vi "Main.vi"() -> ()   [LabVIEW 2020]
doc: "This template is for the Queued Message Handler design pattern.\n\nThe Event Handling Loop generates messages based on user interface actions.\n\nThe Message Handling Loop processes messages generated by the Event Handling Loop, or by other messages. The messages are string values, so new messages can be added easily to the Message Cases case structure in the Message Handling Loop. Each message cluster can also provide an optional value for Message Data, which is a variant that can be converted to whatever message-specific data is required."
uses:
  Newport_FCR100/Libraries/FCR100/Support/Device state -- enum.ctl
  controls/Analysis results -- cluster.ctl
  controls/Abeles-Brewster - Newport UI Data.ctl
  controls/DAQ config parameters -- cluster.ctl
  controls/FCR config parameters -- cluster.ctl
  support/Message Queue/Enqueue Message (Single).vi
  <vilib>/Utility/error.llb/Error Cluster From Error Code.vi
  <vilib>/ErrorRing/Error Ring.xnode
  support/Message Queue/Abeles-Brewster - Newport Message Queue.lvlib
  support/User Event - Stop/Abeles-Brewster - Newport User Event - Stop.lvlib
  Newport_FCR100/Libraries/FCR100/FCR100.lvlib
  NI_DAQ/Libraries/NI DAQ/NI DAQ.lvlib
panel:
  out "Auto?":bool
  out "State 2":T1=enum."Configuration" caption="FCR 2 state"
  out "State 1":T1=enum."Configuration" caption="FCR 1 State"
  out "FCR Connected":bool
  out "DAQ Connected":bool
  in  "Settings":bool
  out "Elapsed time":dbl
  in  "Velocity":dbl=6.0 min=0.001 max=15.0 step=0.001
  in  "Refresh":bool
  in  "Tab Control":T2(tab)
  out "Sensor Value":dbl(slide) caption="Sensor\nValue" scale=0.0..12.0
  out "Angle chart":cluster{"Angle":dbl, "Data":dbl}[](graph)
  in  "Save Data":bool
  in  "File name":string="dato"
  out "Time chart":cluster{"Angle":dbl, "Data":dbl}[](graph)
  in  "Start":bool
  in  "Test time":dbl=6.0
  out "SPR Curve":cluster{"Angle":dbl, "Data":dbl}[](graph)
  in  "q Starting":dbl=40.0 format="%#_g°"
  in  "q Final":dbl=70.0 format="%#_g°"
  in  "Open File":path
  in  "Realizar Análisis":bool
  out "No. de datos":i32
  out "Analysis results":T3 {"Curve width" format="%#.3g°"; "Maximum Intensity" format="%#_gV"; "q Middle" format="%#_g°"; "Minimum Intensity" format="%#_gV"; "qR" format="%#_g°"}
  out "Max":dbl format="%#_g°"
  out "Min":dbl format="%#_g°"
  out "elapsed time 2":dbl
  out "Curr angle":dbl caption="Current Angle P1" format="%#_g°"
  in  "Controls":T4={"AutoMove"={"Move"=FALSE, "Cancel"=FALSE, "Home"=FALSE, "Final Angle P1"=90.0, "Ángulo Final M2"=180.0}, "ManMove"={"Inc platina 1"=FALSE, "Dec platina 1"=FALSE, "Inc platina 2"=FALSE, "Dec platina 2"=FALSE, "Resolution"=1.0}} {"ManMove"."Resolution" min=0.0 max=60.0 step=0.001 format="%#_g°/mov"; "AutoMove"."Ángulo Final M2" min=0.0 max=200.0 step=0.001; "AutoMove"."Final Angle P1" min=0.0 max=250.0 step=0.001 format="%#_g°"}
  in  "Initial Angle P2":dbl=12.0 min=0.0 max=90.0 step=0.001 format="%#_g°"
  in  "Initial Angle P1":dbl=30.0 min=0.0 max=90.0 step=0.001 format="%#_g°"
  in  "Aceleration":dbl=100.0 min=0.001 max=200.0 step=0.001
  in  "Exit":bool
  out "Status":string
  # "CENTRO DE INVESTIGACIONES EN ÓPTICA\nPROGRAM: \nDUAL  STEPPER MOTOR STAGE CONTROL  \n\nDEVELOPMENT BY: M.O. DIEGO TORRES ARMENTA"
  # "q Range"
  # "Conexión platinas\nPlatina 1 -> inf (Dirección 1); Platina 2-> superior (Dirección 2)\nInterfaz USB - RS422-1.8  se cablea entre la computadora y el conector superior correspondiente de platina 1\nCable (azul) FC-CB1 se cablea del conector inferior de platina 1 al conector superior de platina 2.\nSe conectan los eliminadores o fuentes de voltaje a las platinas.\npor último debe de energizar las fuentes de voltaje.\n\n\nConexión tarjeta de adquisición y sensor\n\nConector de sensor-> Amarillo -12V, Rojo +12V, Negro referencia a tierra, Blanco señal.\n\nEl cable blanco del sensor debe ser cableado a la entrada A0 de la tarjeta de adquisición de datos DAQ\nLa DAQ debe ser conectada a la computadora por medio del cable USB correspondiente."
  # "CENTRO DE INVESTIGACIONES EN ÓPTICA\n\nInstrucciones de funcionamiento.\n\n1.- Primero debe asegurar que las conexiones están hechas de manera correcta. (ver apartado conexiones)\n     Platina inferior tiene dirección 1, platina superior tiene dirección 2.\n2.- Se selecciona la velocidad, aceleración, ángulo inicial platina 1 y ángulo inicial platina 2.\n3.- Se ejecuta el programa dando click en el ícono Run, en la parte superior izquierda.\n4.- Aparece una ventana para configurar la dirección de platina a la cual queremos conectarnos, en éste caso seleccionamos 1, además de que en dicha ventana debemos seleccionar la opción (), presionamos aceptar y se da inicio con la ejecución del programa.\n5.- Al ejecutar por primera ocación, plas platinas se moveran de manera automática a posición Home (0 grados), en ejecuciones posteriores se moverán al ángulo inicial predefinido de cada una de las platinas.\n6.- Para ajuste manual debe dar click en los botones Inc++ o Dec -- de cada una de las platinas, el movimiento se realizará la cantidad de grados configurados en el control Resolución, la resolución mínima es de 0.001 y la máxima es de 60, en caso de que las platinas estén en movimiento puede cancelarlo dando click en el botón Cancelar mov.\n7.- Puede mover en cualquier momento las platinas a posición Home (0 grados), presionando el botón Mover a Home.\n8.- Cuando realizó los ajustes necearios en cada platina, se procede a seleccionar el ángulo final de la platina 1,  aquí debe de verificar el ángulo actual de la platina 1  en el indicador correspondiente y debe sumar los grados que desea mover al ángulo actual.\n9.- Una vez configurado se procede a presionar el botón Mover y guardar, entonces las platinas comenzarán su movimiento, guardarán la información en un archivo el cual tiene como nombre la fecha y hora de ejecución del movimiento, adicionalmente se grafica la señal obtenida."
  # "P1"
  # "P2"
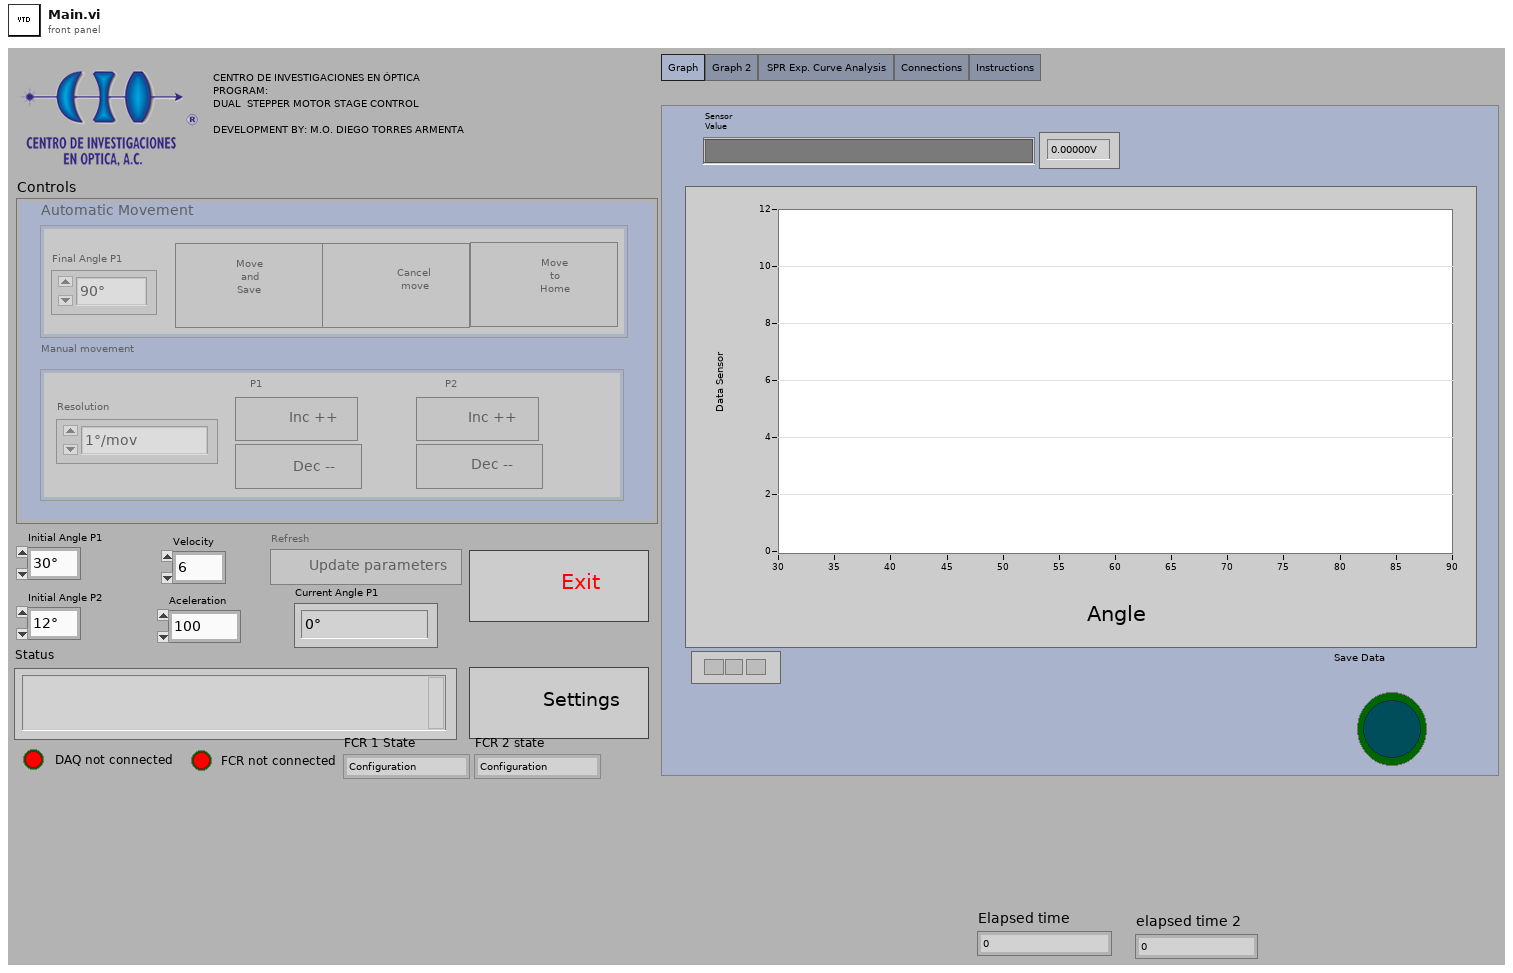
[diagram p1: front panel]
types:
  T1 = typedef "FCR100.lvlib/Device state -- enum.ctl" = enum16{"Not referenced", "Configuration", "Disable", "Ready", "Homing", "Motion"}
  T2 = enum32{"Graph", "Graph 2", "SPR Exp. Curve Analysis ", "Connections", "Instructions"}
  T3 = typedef "Analysis results -- cluster.ctl" = cluster{"q Middle":dbl, "Curve width":dbl, "Maximum Intensity":dbl, "Minimum Intensity":dbl, "qR ":dbl}
  T4 = cluster{"AutoMove":cluster{"Move":bool, "Cancel":bool, "Home":bool, "Final Angle P1":dbl, "Ángulo Final M2":dbl}, "ManMove":cluster{"Inc platina 1":bool, "Dec platina 1":bool, "Inc platina 2":bool, "Dec platina 2":bool, "Resolution":dbl}}
  T5 = typedef "Abeles-Brewster - Newport UI Data.ctl" = cluster{"FCR Mod ID":i32, "DAQ Mod ID":i32, "Status":string, "DAQ config params":T6, "FCR config params":T7, "Connected?":bool, "Home?":bool, "Device state 1":T1, "Device state 2":T1, "Time chart":cluster{"Angle":dbl, "Data":dbl}[], "Angle chart":cluster{"Angle":dbl, "Data":dbl}[], "Initial time":u32}
  T6 = typedef "DAQ config parameters -- cluster.ctl" = cluster{"DAQ Device Name":tag, "Physical channel":tag}
  T7 = typedef "FCR config parameters -- cluster.ctl" = cluster{"VISA resource":refnum<visa-resource-name>, "baud rate":u32, "Acceleration":dbl, "Velocity":dbl, "Initial P1":dbl, "Initial P2":dbl}
  T8 = typedef "FCR100.lvlib/Broadcast Events--cluster.ctl" = cluster{"Module Did Init":refnum<user-event>, "Status Updated":refnum<user-event>, "Error Reported":refnum<user-event>, "Module Did Stop":refnum<user-event>, "Update Module Execution Status":refnum<user-event>, "Device connected":refnum<user-event>, "Connection failed":refnum<user-event>, "Device disconnected":refnum<user-event>, "State reached":refnum<user-event>, "Home reached":refnum<user-event>}
  T9 = typedef "NI DAQ.lvlib/Broadcast Events--cluster.ctl" = cluster{"Module Did Init":refnum<user-event>, "Status Updated":refnum<user-event>, "Error Reported":refnum<user-event>, "Module Did Stop":refnum<user-event>, "Update Module Execution Status":refnum<user-event>, "Digital data acquired":refnum<user-event>, "Device connected":refnum<user-event>, "Connection failed":refnum<user-event>, "Analog data acquired":refnum<user-event>}
  T10 = typedef "Abeles-Brewster - Newport Message Queue.lvlib/All Message Queues.ctl" = cluster{"UI":refnum<queue>}
  T11 = enum8{"Enabled", "Disabled", "Disabled and Grayed Out"}
  T12 = enum16{"All", "DO task", "DI task", "AO task", "AI task"}
  T13 = cluster{"input terminal configuration":i32, "minimum value":dbl, "maximum value":dbl}
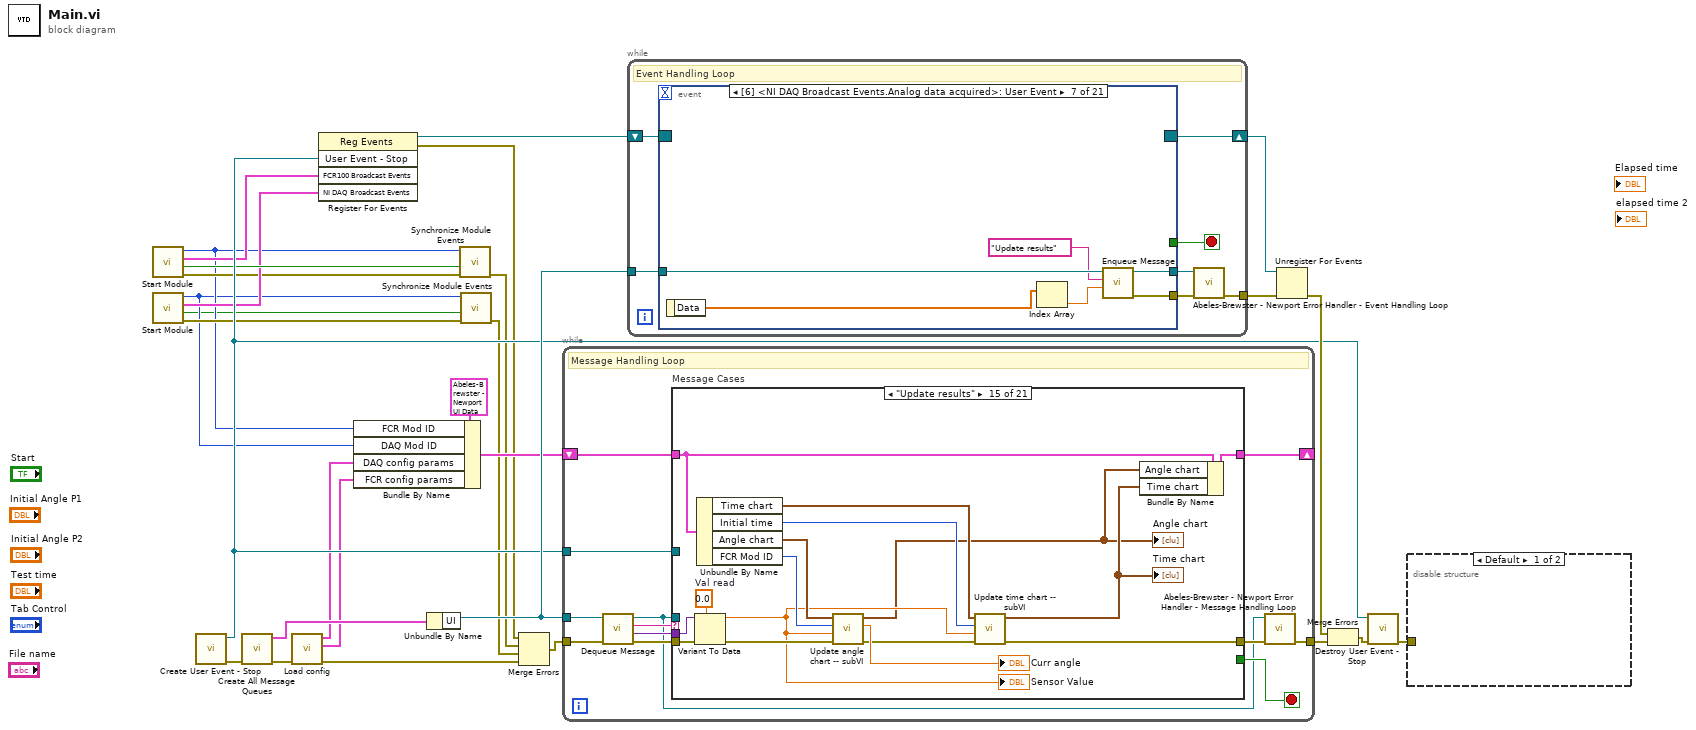
[diagram p0: block diagram]
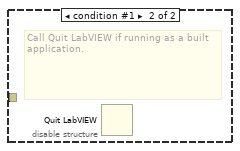
[diagram p2: hidden frame]
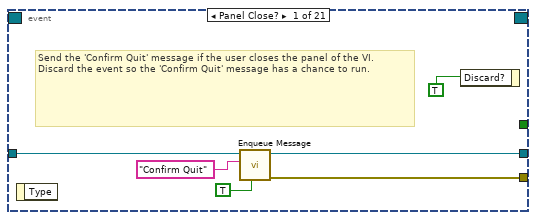
[diagram p3: hidden frame]
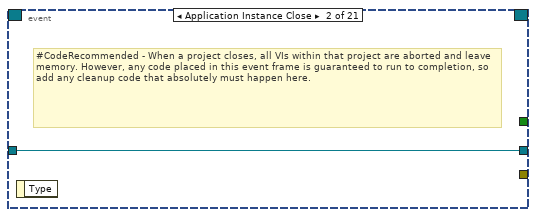
[diagram p4: hidden frame]
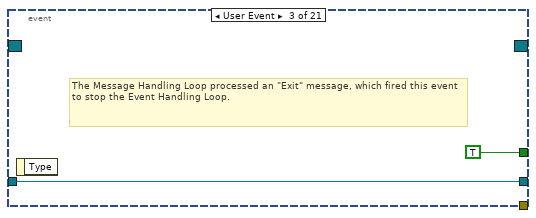
[diagram p5: hidden frame]
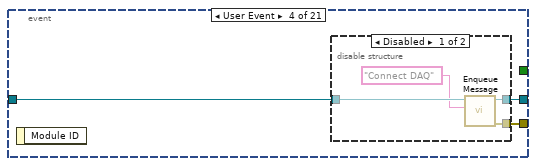
[diagram p6: hidden frame]
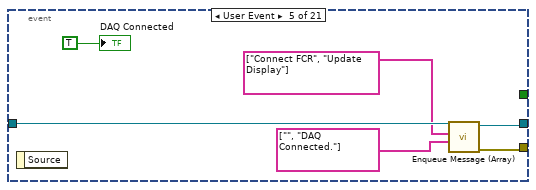
[diagram p8: hidden frame]
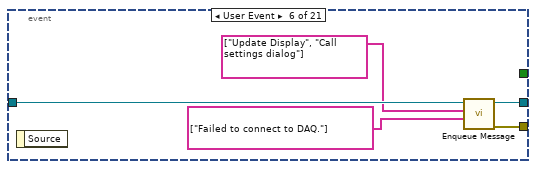
[diagram p9: hidden frame]
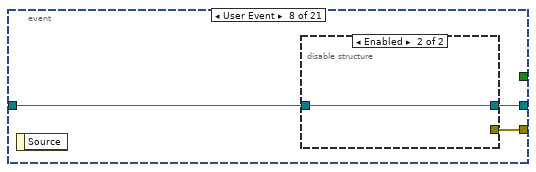
[diagram p10: hidden frame]
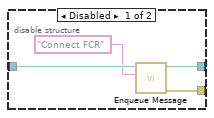
[diagram p11: hidden frame]
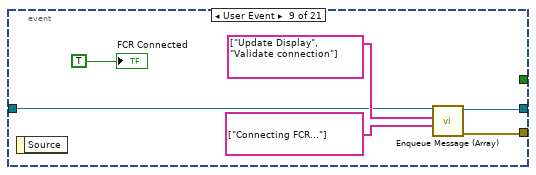
[diagram p12: hidden frame]
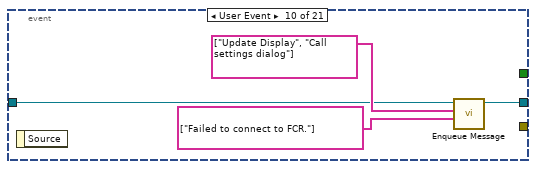
[diagram p13: hidden frame]
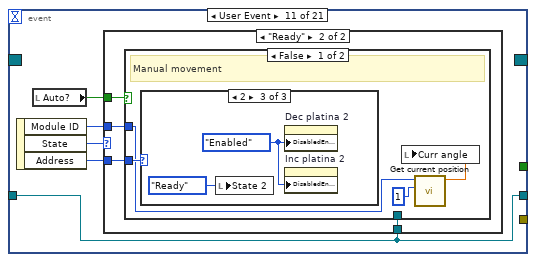
[diagram p14: hidden frame]
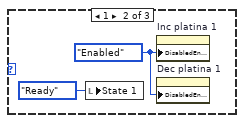
[diagram p17: hidden frame]
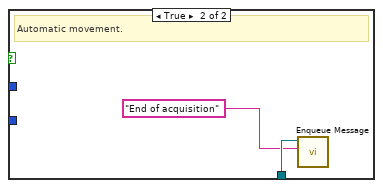
[diagram p18: hidden frame]
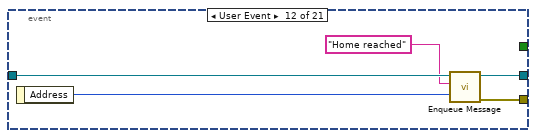
[diagram p19: hidden frame]
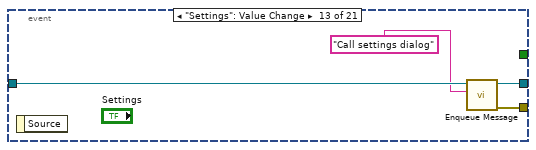
[diagram p20: hidden frame]
diagram:
  n1 = call "Start Module.vi"() -> ("error out"=w13:errorcluster, "Wait for Event Sync?"=w16:bool, "FCR100 Broadcast Events"=w17:T8, "Module ID"=w7:i32)  [unwired: 8 in]
  n2 = call "Start Module.vi"() -> ("error out"=w15:errorcluster, "Wait for Event Sync?"=w5:bool, "NI DAQ Broadcast Events"=w14:T9, "Module ID"=w6:i32)  [unwired: 8 in]
  n3 = call "Create User Event - Stop.vi"() -> ("error out"=w26:errorcluster, "User Event - Stop"=w19:refnum<user-event>)  [unwired: 10 in]
  n4 = call "Create All Message Queues.vi"("error in (no error)"=w26) -> ("error out"=w4:errorcluster, "Message Queues out"=w29:T10)  [unwired: 9 in]
  n5 = call "Load config.vi"("error in (no error)"=w4) -> ("DAQ config params"=w2:T6, "FCR config params"=w1:T7, "error out"=w3:errorcluster)  [unwired: 7 in]
  n6 = register-events(w19, w17, w14) -> (reference out=w20:refnum<event-registration>, error out=w8:errorcluster)  [unwired: 2 in]
  n7 = Bundle By Name(cluster=T5 {"FCR Mod ID"=0, "DAQ Mod ID"=0, "Status"="", "DAQ config params"={"DAQ Device Name"="Dev2", "Physical channel"=""}, "FCR config params"={"VISA resource"="", "baud rate"=9600, "Acceleration"=0.0, "Velocity"=0.0, "Initial P1"=0.0, "Initial P2"=0.0}, "Connected?"=FALSE, "Home?"=FALSE, "Device state 1"=enum."Configuration", "Device state 2"=enum."Configuration", "Time chart"=[], "Angle chart"=[], "Initial time"=0} ("Data Cluster"), "FCR Mod ID"=w7, "DAQ Mod ID"=w6, "DAQ config params"=w2, "FCR config params"=w1) -> (w11:T5)
  n8 = Unbundle By Name(w29) -> ("UI"=w27:refnum<queue>)
  n9 = call "Synchronize Module Events.vi"("error in"=w13, "Wait for Event Sync?"=w16, "Module ID in"=w7) -> ("error out"=w9:errorcluster)  [unwired: 7 in, 1 out]
  n10 = call "Synchronize Module Events.vi"("error in"=w15, "Wait for Event Sync?"=w5, "Module ID in"=w6) -> ("error out"=w10:errorcluster)  [unwired: 7 in, 1 out]
  n11 = Merge Errors(w8, w9, w10, w3) -> (w18:errorcluster)
  n12 = while {
    tunnel: w27 -> [w33]
    shift-right: [w40] -> _
    shift-left: w11 -> [w41]
    tunnel: w19 -> [w38]
    tunnel: w18 -> [w37]
    tunnel: [w32] -> w28
    stop <- w39 stop-if-true
    # "Message Handling Loop"
    n13 = call "Dequeue Message.vi"("error in (no error)"=w37, "Message Queue"=w33) -> ("error out"=w36:errorcluster, "Message Data"=w34:variant, "Message"=w35:string, "dup Message Queue"=w30:refnum<queue>)  [unwired: 6 in]
    n14 = case "Message Cases" shown="\"Update results\"" w35 {
      selector: w35 -> [_ _ _ _ _ _ _ _ _ _ _ _ _ _ _ _ _ _ _ _ w392]
      tunnel: w30 -> [w58 _ w84 w102 _ _ w125 _ w175 _ _ _ w270 w279 _ _ _ _ w363 w391 _]
      tunnel: w36 -> [w47 w76 w81 w105 w117 w123 w134 w160 w168 w180 w203 w258 w273 w285 w308 w323 w328 w360 w367 w386 _]
      tunnel: [w60 w77 w85 w104 w111 w122 w133 w158 w176 w185 w196 w256 w271 w282 w295 w311 w326 w354 w365 w389 w393] -> w31
      tunnel: w41 -> [w51 w63 w87 w106 w116 w121 w127 w153 w167 w184 w193 w249 w261 w284 w302 w324 w331 w359 w366 w382 w394]
      tunnel: [w50 w61 w89 w106 w116 w121 w126 w152 w174 w183 w192 w248 w259 w284 w301 w324 w331 w359 w366 w382 w394] -> w40
      tunnel: [_ _ _ _ _ _ _ _ _ _ _ _ _ _ _ _ _ _ _ TRUE _] -> w39
      tunnel: w34 -> [_ w75 _ _ _ _ _ _ _ _ w202 _ _ _ w306 w322 _ w358 _ w383 _]
      tunnel: w38 -> [_ _ _ _ _ _ _ _ _ _ _ _ _ _ _ _ _ _ _ w388 _]
      frame "Initialize" {
        w49 = FALSE ("Connected?")
        w56 = T11."Disabled and Grayed Out" ("Disabled")
        # "Initialize - All initialization work should take place in this message, since other loops can potentially enqueue messages that execute immediately after this one."
        n15 = control-ref of="This VI"() -> (w48:refnum<vi>)
        n16 = Unbundle By Name(w51) -> ("FCR config params.Acceleration"=w55:dbl, "FCR config params.Velocity"=w54:dbl, "FCR config params.Initial P1"=w53:dbl, "FCR config params.Initial P2"=w52:dbl)
        n17 = invoke on="Invoke Node" class="VI" method="Default Vals.Reinit All"(reference=w48, error in=w47) -> (reference out=w43:refnum<vi>, error out=w44:errorcluster)  [unwired: 1 in, 1 out]
        n18 = property on="Aceleration" class="DigNum (strict)"("Value"=w55) -> ()  [unwired: 2 in, 2 out]
        n19 = property on="Velocity" class="DigNum (strict)"("Value"=w54) -> ()  [unwired: 2 in, 2 out]
        n20 = property on="Initial P1" class="DigNum (strict)"("Value"=w53) -> ()  [unwired: 2 in, 2 out]
        n21 = property on="Initial P2" class="DigNum (strict)"("Value"=w52) -> ()  [unwired: 2 in, 2 out]
        n22 = invoke on="Invoke Node" class="VI" method="FP.Center"(reference=w43, error in=w44) -> (error out=w42:errorcluster)  [unwired: 1 in, 2 out]
        n23 = Bundle By Name(cluster=w51, "Connected?"=w49, "Home?"=w49, "Angle chart"=cluster{"Angle":dbl, "Data":dbl}[] [], "Time chart"=cluster{"Angle":dbl, "Data":dbl}[] []) -> (w50:T5)
        n24 = property on="AutoMove" class="Clust"("DisabledEnum"=w56) -> ()  [unwired: 2 in, 2 out]
        n25 = property on="ManMove" class="Clust"("DisabledEnum"=w56) -> ()  [unwired: 2 in, 2 out]
        n26 = property on="Refresh" class="Bool"("DisabledEnum"=w56) -> ()  [unwired: 2 in, 2 out]
        n27 = call-poly "Enqueue Message.vi"("error in (no error)"=w42, "Message Data Array"=string[] ["Initializing..."] ("Message"), "Message Array"=string[] ["Update Display", "Connect DAQ"] ("Message"), "Message Queue"=w58) -> ("error out"=w60:errorcluster)  [unwired: 6 in, 1 out]
      }
      frame "Update Display" {
        # "Update Display - Convert the message data to a string to display in the Data Display indicator."
        n28 = Variant To Data(error in=w76, type="", Variant=w75) -> (data=w68:string, error out=w66:errorcluster)
        n29 = Unbundle By Name(w63) -> ("Status"=w69:string)
        n30 = Get Date/Time In Seconds() -> (seconds since 1Jan1904=w72:timestamp)
        n31 = Format Date/Time String(time format string (%c)="%d/%m/%y %H:%M:%S%3u", seconds (now)=w72) -> (date/time string=w70:string)  [unwired: 1 in]
        n32 = Format Into String(format string="%s: %s\\n", initial string=w69, error in=w66, w70, w68) -> (resulting string=w62:string, error out=w67:errorcluster)
        "Status" <- w62
        n33 = property on="Status" class="Str"(error in=w67, "Text.Scroll Position"=u32 2000) -> (error out=w65:errorcluster)  [unwired: 1 in, 1 out]
        n34 = Bundle By Name(cluster=w63, "Status"=w62) -> (w61:T5)
        n35 = Merge Errors(w65) -> (w77:errorcluster)
      }
      frame "Call settings dialog" {
        n36 = Unbundle By Name(w87) -> ("DAQ config params"=w88:T6, "FCR config params"=w78:T7, "FCR Mod ID"=w80:i32)
        n37 = call "Disconnect.vi"("error in"=w81, "Module ID"=w80) -> ("error out"=w79:errorcluster)  [unwired: 9 in]
        n38 = call "Config dialog.vi"("error in (no error)"=w79, "FCR config params in"=w78, "DAQ config params in"=w88) -> ("error out"=w90:errorcluster, "Cancelled?"=w83:bool, "FCR config params out"=w82:T7, "DAQ config params out"=w86:T6)  [unwired: 5 in]
        n39 = case shown="False" w83 {
          tunnel: w90 -> [w94 w100]
          tunnel: w87 -> [w99 w101]
          tunnel: [w98 w101] -> w89
          tunnel: w86 -> [w92 _]
          tunnel: [w97 w100] -> w85
          tunnel: w84 -> [w96 _]
          tunnel: w82 -> [w91 _]
          frame False {
            # "Dialog not cancelled. Save and apply config."
            n40 = Bundle By Name(cluster=w99, "DAQ config params"=w92, "FCR config params"=w91) -> (w98:T5)
            n41 = call "Write config.vi"("error in (no error)"=w94, "FCR config params"=w91, "DAQ config params"=w92) -> ("error out"=w93:errorcluster)  [unwired: 8 in]
            n42 = call-poly "Enqueue Message.vi"("error in (no error)"=w93, "Message"="Apply configuration", "Message Queue"=w96) -> ("error out"=w97:errorcluster)  [unwired: 7 in, 1 out]
          }
          frame True {
            # "Dialog was cancelled. Do nothing."
          }
        }
      }
      frame "Apply configuration" {
        n43 = call-poly "Enqueue Message.vi"("error in (no error)"=w105, "Message Array"=string[] ["Connect DAQ", "Connect FCR"] ("Message"), "Message Queue"=w102) -> ("error out"=w104:errorcluster)  [unwired: 7 in, 1 out]
      }
      frame "Connect DAQ" {
        w115 = T13 {"input terminal configuration"=10083, "minimum value"=-10.0, "maximum value"=10.0}  # Config params
        n44 = Unbundle By Name(w116) -> ("DAQ Mod ID"=w108:i32, "DAQ config params.Physical channel"=w114:tag, "DAQ config params.DAQ Device Name"=w110:tag)
        n45 = call "Set device ID.vi"("error in"=w117, "Device ID"=w110, "Module ID"=w108) -> ("error out"=w109:errorcluster)  [unwired: 8 in]
        n46 = call "Validate connection.vi"("error in"=w109, "Module ID"=w108) -> ("error out"=w107:errorcluster)  [unwired: 7 in, 2 out]
        n47 = call "Create AI channel.vi"("Config params"=w115, "error in"=w107, "Channel name"="Sensor", "Physical channel"=w114, "Module ID"=w108) -> ("error out"=w112:errorcluster)  [unwired: 6 in]
        n48 = call "Start task.vi"("error in"=w112, "Module ID"=w108) -> ("error out"=w111:errorcluster)  [unwired: 9 in]
      }
      frame "Connect FCR" {
        n49 = Unbundle By Name(w121) -> ("FCR Mod ID"=w120:i32, "FCR config params.VISA resource"=w119:refnum<visa-resource-name>, "FCR config params.baud rate"=w118:u32)
        n50 = call "Connect wihtout dialog.vi"("error in"=w123, "baud rate"=w118, "VISA resource"=w119, "Module ID"=w120) -> ("error out"=w122:errorcluster)  [unwired: 7 in]
      }
      frame "Validate connection" {
        n51 = Unbundle By Name(w127) -> ("FCR Mod ID"=w124:i32, "Connected?"=w129:bool)
        n52 = local read "DAQ Connected"() -> (w131:bool)
        n53 = local read "FCR Connected"() -> (w130:bool)
        n54 = Not(x=w129) -> (.not. x?=w128:bool)
        n55 = Compound Arithmetic op=AND(w128, w131, w130) -> (w132:bool)
        n56 = case shown="True" w132 {
          tunnel: w134 -> [w136 w144]
          tunnel: [w136 w147] -> w133
          tunnel: w127 -> [w135 w150]
          tunnel: [w135 w148] -> w126
          tunnel: w125 -> [_ w146]
          tunnel: w124 -> [_ w139]
          frame False {
          }
          frame True {
            w143 = Device_state_--_enum."Not referenced" ("State")
            # "Reset both controllers and send home afterwards."
            n57 = local read "Aceleration"() -> (w138:dbl)
            n58 = local read "Velocity"() -> (w137:dbl)
            n59 = call "Reset devices.vi"("error in (no error)"=w144, "FCR Mod ID"=w139) -> ("error out"=w141:errorcluster)  [unwired: 9 in]
            n60 = call "Update FCR parameters -- subVI.vi"("error in (no error)"=w141, "Velocity"=w137, "Aceleration"=w138, "FCR Mod ID"=w139) -> ("error out"=w140:errorcluster)  [unwired: 7 in]
            n61 = Bundle By Name(cluster=w150, "Connected?"=TRUE, "Device state 1"=w143, "Device state 2"=w143) -> (w148:T5)
            n62 = local write "State 2"(w143) -> ()
            n63 = local write "State 1"(w143) -> ()
            n64 = call-poly "Enqueue Message.vi"("error in (no error)"=w140, "Message Data Array"=string[] ["FCR Connected. Homing..."] ("Message"), "Message Array"=string[] ["Update display", "Home"] ("Message"), "Message Queue"=w146) -> ("error out"=w147:errorcluster)  [unwired: 6 in, 1 out]
          }
        }
      }
      frame "Home" {
        w151 = Device_state_--_enum."Homing" ("Device state 1")
        w154 = T11."Disabled and Grayed Out" ("Disabled")
        n65 = Unbundle By Name(w153) -> ("FCR Mod ID"=w157:i32)
        n66 = call "Send home.vi"("error in (no error)"=w160, "FCR Mod ID"=w157) -> ("error out"=w159:errorcluster)  [unwired: 8 in, 1 out]
        n67 = call "Continuously check state.vi"("error in"=w159, "Desired state"=Device_state_--_enum."Ready", "Address"=u8 2, "Module ID"=w157) -> ("error out"=w158:errorcluster)  [unwired: 7 in]
        n68 = Bundle By Name(cluster=w153, "Device state 1"=w151, "Device state 2"=w151) -> (w152:T5)
        n69 = local write "State 2"(w151) -> ()
        n70 = local write "State 1"(w151) -> ()
        n71 = property on="AutoMove" class="Clust"("DisabledEnum"=w154) -> ()  [unwired: 2 in, 2 out]
        n72 = property on="ManMove" class="Clust"("DisabledEnum"=w154) -> ()  [unwired: 2 in, 2 out]
        n73 = property on="Refresh" class="Bool"("DisabledEnum"=w154) -> ()  [unwired: 2 in, 2 out]
      }
      frame "Home reached" {
        w161 = 2.0 ("Position")
        w172 = Device_state_--_enum."Ready" ("Device state 1")
        w173 = T11."Enabled" ("Disabled")
        n74 = Unbundle By Name(w167) -> ("FCR Mod ID"=w164:i32)
        n75 = call "Move relative.vi"("error in"=w168, "Position"=w161, "Address"=u8 1, "Module ID"=w164) -> ("error out"=w162:errorcluster)  [unwired: 7 in]
        n76 = call "Move relative.vi"("error in"=w162, "Position"=w161, "Address"=u8 2, "Module ID"=w164) -> ("error out"=w165:errorcluster)  [unwired: 7 in]
        n77 = property on="AutoMove" class="Clust"("DisabledEnum"=w173) -> ()  [unwired: 2 in, 2 out]
        n78 = property on="ManMove" class="Clust"("DisabledEnum"=w173) -> ()  [unwired: 2 in, 2 out]
        n79 = property on="Refresh" class="Bool"("DisabledEnum"=w173) -> ()  [unwired: 2 in, 2 out]
        n80 = Bundle By Name(cluster=w167, "Home?"=TRUE, "Device state 1"=w172, "Device state 2"=w172) -> (w174:T5)
        n81 = local write "State 2"(w172) -> ()
        n82 = local write "State 1"(w172) -> ()
        n83 = call-poly "Enqueue Message.vi"("error in (no error)"=w165, "Message Data"="Home reached." ("Message"), "Message"="Update Display", "Message Queue"=w175) -> ("error out"=w176:errorcluster)  [unwired: 6 in, 1 out]
      }
      frame "Stop movement" {
        n84 = Unbundle By Name(w184) -> ("FCR Mod ID"=w178:i32)
        n85 = call "Stop checking state.vi"("error in"=w180, "Address"=u8 1, "Module ID"=w178) -> ("error out"=w179:errorcluster)  [unwired: 8 in]
        n86 = call "Stop movement.vi"("error in"=w179, "Address"=u8 0, "Module ID"=w178) -> ("error out"=w189:errorcluster)  [unwired: 8 in]
        n87 = call "Get state.vi"("error in"=w189, "Address"=u8 1, "Module ID"=w178) -> ("error out"=w188:errorcluster, "Device state"=w181:T1)  [unwired: 6 in, 1 out]
        "State 1" <- w181
        n88 = call "Get state.vi"("error in"=w188, "Address"=u8 2, "Module ID"=w178) -> ("error out"=w185:errorcluster, "Device state"=w182:T1)  [unwired: 6 in, 1 out]
        "State 2" <- w182
        n89 = Bundle By Name(cluster=w184, "Device state 1"=w181, "Device state 2"=w182) -> (w183:T5)
        n90 = local write "State 1"(w181) -> ()
        n91 = local write "State 2"(w182) -> ()
      }
      frame "Manual move" {
        n92 = Variant To Data(error in=w203, type=refnum<vi> refnum ("CtlRef"), Variant=w202) -> (data=w200:refnum<vi>, error out=w199:errorcluster)
        n93 = Unbundle By Name(w193) -> ("FCR Mod ID"=w194:i32)
        n94 = property class="Bool"(reference=w200, error in=w199) -> (error out=w197:errorcluster, "Label.Text"=w198:string)  [unwired: 1 out]
        n95 = property on="Resolution" class="DigNum (strict)"() -> ("Value"=w195:dbl)  [unwired: 2 in, 2 out]
        n96 = case shown="\"Dec platina 2\"" w198 {
          tunnel: w197 -> [w205 w214 w224 w233 w243]
          tunnel: [w205 w209 w218 w228 w238] -> w196
          tunnel: w195 -> [_ w213 w223 w232 w242]
          tunnel: w194 -> [_ w208 w217 w227 w237]
          tunnel: [TRUE ("Home?") _ _ _ _] -> w191
          frame Default {
          }
          frame "Inc platina 1" {
            w212 = T11."Disabled and Grayed Out" ("Disabled")
            w207 = u8 1 ("Numeric")
            n97 = call "Move relative.vi"("error in"=w214, "Position"=w213, "Address"=w207, "Module ID"=w208) -> ("error out"=w210:errorcluster)  [unwired: 7 in]
            n98 = local write "State 1"(Device_state_--_enum."Motion" ("State 1")) -> ()
            n99 = property on="Inc platina 1" class="Bool"("DisabledEnum"=w212) -> ()  [unwired: 2 in, 2 out]
            n100 = property on="Dec platina 1" class="Bool"("DisabledEnum"=w212) -> ()  [unwired: 2 in, 2 out]
            n101 = call "Continuously check state.vi"("error in"=w210, "Desired state"=Device_state_--_enum."Ready", "Address"=w207, "Module ID"=w208) -> ("error out"=w209:errorcluster)  [unwired: 7 in]
          }
          frame "Dec platina 1" {
            w221 = T11."Disabled and Grayed Out" ("Disabled")
            w216 = u8 1 ("Numeric")
            n102 = Negate(x=w223) -> (-x=w222:dbl)
            n103 = call "Move relative.vi"("error in"=w224, "Position"=w222, "Address"=w216, "Module ID"=w217) -> ("error out"=w219:errorcluster)  [unwired: 7 in]
            n104 = local write "State 1"(Device_state_--_enum."Motion" ("State 1")) -> ()
            n105 = call "Continuously check state.vi"("error in"=w219, "Desired state"=Device_state_--_enum."Ready", "Address"=w216, "Module ID"=w217) -> ("error out"=w218:errorcluster)  [unwired: 7 in]
            n106 = property on="Dec platina 1" class="Bool"("DisabledEnum"=w221) -> ()  [unwired: 2 in, 2 out]
            n107 = property on="Inc platina 1" class="Bool"("DisabledEnum"=w221) -> ()  [unwired: 2 in, 2 out]
          }
          frame "Inc platina 2" {
            w231 = T11."Disabled and Grayed Out" ("Disabled")
            w226 = u8 2 ("Numeric")
            n108 = call "Move relative.vi"("error in"=w233, "Position"=w232, "Address"=w226, "Module ID"=w227) -> ("error out"=w229:errorcluster)  [unwired: 7 in]
            n109 = local write "State 2"(Device_state_--_enum."Motion" ("State 1")) -> ()
            n110 = call "Continuously check state.vi"("error in"=w229, "Desired state"=Device_state_--_enum."Ready", "Address"=w226, "Module ID"=w227) -> ("error out"=w228:errorcluster)  [unwired: 7 in]
            n111 = property on="Dec platina 2" class="Bool"("DisabledEnum"=w231) -> ()  [unwired: 2 in, 2 out]
            n112 = property on="Inc platina 2" class="Bool"("DisabledEnum"=w231) -> ()  [unwired: 2 in, 2 out]
          }
          frame "Dec platina 2" {
            w240 = T11."Disabled and Grayed Out" ("Disabled")
            w236 = u8 1 ("Numeric")
            n113 = Negate(x=w242) -> (-x=w241:dbl)
            n114 = call "Move relative.vi"("error in"=w243, "Position"=w241, "Address"=w236, "Module ID"=w237) -> ("error out"=w239:errorcluster)  [unwired: 7 in]
            n115 = local write "State 2"(Device_state_--_enum."Motion" ("State 1")) -> ()
            n116 = call "Continuously check state.vi"("error in"=w239, "Desired state"=Device_state_--_enum."Ready", "Address"=w236, "Module ID"=w237) -> ("error out"=w238:errorcluster)  [unwired: 7 in]
            n117 = property on="Dec platina 2" class="Bool"("DisabledEnum"=w240) -> ()  [unwired: 2 in, 2 out]
            n118 = property on="Inc platina 2" class="Bool"("DisabledEnum"=w240) -> ()  [unwired: 2 in, 2 out]
          }
        }
        n119 = Bundle By Name(cluster=w193, "Home?"=w191) -> (w192:T5)
      }
      frame "Start aqcuisition" {
        w246 = cluster{"Angle":dbl, "Data":dbl}[] [] ("Time chart")
        w247 = cluster{"Angle":dbl, "Data":dbl}[] [] ("Angle chart")
        w253 = Device_state_--_enum."Motion" ("State 1")
        w254 = T11."Disabled and Grayed Out" ("Disabled")
        n120 = Unbundle By Name(w249) -> ("DAQ Mod ID"=w250:i32, "FCR Mod ID"=w251:i32)
        n121 = Unbundle By Name("Controls") -> ("AutoMove.Final Angle P1"=w252:dbl)
        n122 = local write "State 1"(w253) -> ()
        n123 = local write "State 2"(w253) -> ()
        n124 = property on="ManMove" class="Clust"("DisabledEnum"=w254) -> ()  [unwired: 2 in, 2 out]
        n125 = property on="Move" class="Bool"("DisabledEnum"=w254) -> ()  [unwired: 2 in, 2 out]
        n126 = property on="Refresh" class="Bool"("DisabledEnum"=w254) -> ()  [unwired: 2 in, 2 out]
        n127 = property on="Cancel" class="Bool"("DisabledEnum"=T11."Enabled" ("Disabled")) -> ()  [unwired: 2 in, 2 out]
        n128 = property on="Home" class="Bool"("DisabledEnum"=w254) -> ()  [unwired: 2 in, 2 out]
        n129 = call "Setup and start acquisition.vi"("error in (no error)"=w258, "Final Angle P1"=w252, "FCR Mod ID"=w251, "DAQ Mod ID"=w250) -> ("error out"=w256:errorcluster)  [unwired: 7 in]
        n130 = Tick Count (ms)() -> (millisecond timer value=w245:u32)
        n131 = Bundle By Name(cluster=w249, "Initial time"=w245, "Angle chart"=w247, "Time chart"=w246) -> (w248:T5)
        n132 = property on="Time chart" class="XYGraph (strict)"("Value"=w246) -> ()  [unwired: 2 in, 2 out]
        n133 = property on="Angle chart" class="XYGraph (strict)"("Value"=w247) -> ()  [unwired: 2 in, 2 out]
        "Auto?" <- TRUE ("Auto?")
      }
      frame "Update FCR parameters" {
        n134 = Unbundle By Name(w261) -> ("DAQ config params"=w265:T6, "FCR config params"=w264:T7, "FCR Mod ID"=w272:i32)
        n135 = call "Update FCR parameters -- subVI.vi"("error in (no error)"=w273, "Velocity"="Velocity", "Aceleration"="Aceleration", "FCR Mod ID"=w272) -> ("error out"=w267:errorcluster)  [unwired: 7 in]
        n136 = Bundle By Name(cluster=w264, "Acceleration"="Aceleration", "Velocity"="Velocity") -> (w260:T7)
        n137 = Bundle By Name(cluster=w261, "FCR config params"=w260) -> (w259:T5)
        n138 = call "Write config.vi"("error in (no error)"=w267, "FCR config params"=w260, "DAQ config params"=w265) -> ("error out"=w266:errorcluster)  [unwired: 8 in]
        n139 = call-poly "Enqueue Message.vi"("error in (no error)"=w266, "Message Data"="Acceleration and velocity updated." ("Message"), "Message"="Update Display", "Message Queue"=w270) -> ("error out"=w271:errorcluster)  [unwired: 6 in, 1 out]
      }
      frame "End of acquistion" {
        w286 = T11."Enabled" ("Disabled")
        n140 = Unbundle By Name(w284) -> ("Angle chart"=w275:cluster{"Angle":dbl, "Data":dbl}[], "DAQ Mod ID"=w283:i32)
        n141 = local write "Auto?"(FALSE ("Auto?")) -> ()
        n142 = call "Stop continuous acquisition.vi"("error in"=w285, "Module ID"=w283) -> ("error out"=w277:errorcluster)  [unwired: 9 in]
        n143 = case shown="True" "Save Data" {
          tunnel: w277 -> [w288 w292]
          tunnel: w275 -> [_ w291]
          tunnel: [w288 w290] -> w274
          frame False {
          }
          frame True {
            n144 = call "Save file.vi"("error in (no error)"=w292, "prompt"="Angle vs I", "Angle chart"=w291) -> ("error out"=w290:errorcluster)  [unwired: 8 in]
          }
        }
        n145 = property on="ManMove" class="Clust"("DisabledEnum"=w286) -> ()  [unwired: 2 in, 2 out]
        n146 = property on="Cancel" class="Bool"("DisabledEnum"=T11."Disabled and Grayed Out" ("Disabled")) -> ()  [unwired: 2 in, 2 out]
        n147 = property on="Move" class="Bool"("DisabledEnum"=w286) -> ()  [unwired: 2 in, 2 out]
        n148 = property on="Home" class="Bool"("DisabledEnum"=w286) -> ()  [unwired: 2 in, 2 out]
        n149 = property on="Refresh" class="Bool"("DisabledEnum"=w286) -> ()  [unwired: 2 in, 2 out]
        n150 = call-poly "Enqueue Message.vi"("error in (no error)"=w274, "Message Data"="Acquisition complete." ("Message"), "Message"="Update Display", "Message Queue"=w279) -> ("error out"=w282:errorcluster)  [unwired: 6 in, 1 out]
      }
      frame "Update results" {
        w305 = 0.0  # Val read
        n151 = Variant To Data(error in=w308, type=w305, Variant=w306) -> (data=w298:dbl, error out=w300:errorcluster)
        "Sensor Value" <- w298
        n152 = Unbundle By Name(w302) -> ("Time chart"=w304:cluster{"Angle":dbl, "Data":dbl}[], "Initial time"=w307:u32, "Angle chart"=w303:cluster{"Angle":dbl, "Data":dbl}[], "FCR Mod ID"=w299:i32)
        n153 = call "Update angle chart -- subVI.vi"("error in (no error)"=w300, "Val read"=w298, "FCR Mod ID"=w299, "Angle chart in"=w303) -> ("error out"=w296:errorcluster, "Position"=→"Curr angle":dbl, "Angle chart out"=w293:cluster{"Angle":dbl, "Data":dbl}[])  [unwired: 5 in]
        "Angle chart" <- w293
        n154 = call "Update time chart -- subVI.vi"("error in (no error)"=w296, "Val read"=w298, "Initial time"=w307, "Time chart in"=w304) -> ("error out"=w295:errorcluster, "Time chart out"=w294:cluster{"Time":dbl, "Data":dbl}[])  [unwired: 6 in]
        "Time chart" <- w294
        n155 = Bundle By Name(cluster=w302, "Angle chart"=w293, "Time chart"=w294) -> (w301:T5)
      }
      frame "Update range" {
        n156 = Variant To Data(error in=w323, type=path "", Variant=w322) -> (data=w319:path, error out=w320:errorcluster)
        n157 = Open/Create/Replace File(file path (use dialog)=w319, error in=w320, access (0:read/write)=enum16{"read/write", "read-only", "write-only"}."read-only") -> (refnum out=w316:refnum<file>, error out=w317:errorcluster)  [unwired: 3 in, 1 out]
        n158 = Read from Text File(file (use dialog)=w316, error in=w317) -> (refnum out=w315:refnum<file>, text=w313:string, error out=w314:errorcluster)  [unwired: 2 in, 1 out]
        n159 = Close File(refnum=w315, error in=w314) -> (error out=w312:errorcluster)  [unwired: 1 out]
        n160 = call "Get angle range.vi"("error in (no error)"=w312, "String"=w313) -> ("error out"=w311:errorcluster, "Min"=→"Min":dbl, "Max"=→"Max":dbl)  [unwired: 7 in]
      }
      frame "Analyze data" {
        n161 = Open/Create/Replace File(file path (use dialog)="Open File", error in=w328, access (0:read/write)=enum16{"read/write", "read-only", "write-only"}."read-only") -> (refnum out=w325:refnum<file>, error out=w327:errorcluster)  [unwired: 3 in, 1 out]
        n162 = case shown="No Error" w327 {
          selector: w327 -> [w345 w348 w351]
          tunnel: [w339 w346 w353] -> w326
          tunnel: w325 -> [w344 _ _]
          frame No Error {
            n163 = Read from Text File(file (use dialog)=w344, error in=w345) -> (refnum out=w342:refnum<file>, text=w341:string, error out=w343:errorcluster)  [unwired: 2 in, 1 out]
            n164 = Close File(refnum=w342, error in=w343) -> (error out=w340:errorcluster)  [unwired: 1 out]
            n165 = call "Import data --subVI.vi"("error in (no error)"=w340, "String"=w341) -> ("error out"=w338:errorcluster, "Array"=w335:cluster{"Angle":dbl, "Data":dbl}[])  [unwired: 8 in]
            n166 = call "Analyze SPR data -- subVI.vi"("error in (no error)"=w338, "q Final"="q Final", "q Starting"="q Starting", "Data"=w335) -> ("error out"=w339:errorcluster, "No. de datos"=→"No. de datos":i32, "Analysis results"=→"Analysis results":T3, "SPR curve"=→"SPR Curve":cluster{"Angle":dbl, "Data":dbl}[])  [unwired: 4 in]
          }
          frame Error {
            n167 = call <vilib>:"Clear Errors.vi"("error in (no error)"=w348) -> ("error out"=w346:errorcluster)  [unwired: 5 in, 1 out]
            n168 = One Button Dialog(message="Filepath is not  valid or empty. Please select a valid path.") -> ()  [unwired: 1 in, 1 out]
          }
          frame Default {
            n169 = Unbundle By Name(w351) -> ("code"=w350:i32)
            n170 = call <vilib>:"Clear Errors.vi"("error in (no error)"=w351) -> ("error out"=w353:errorcluster)  [unwired: 5 in, 1 out]
            n171 = Format Into String(format string="Unknown error. Error code: %d." ("message"), w350) -> (resulting string=w349:string)  [unwired: 2 in, 1 out]
            n172 = One Button Dialog(message=w349) -> ()  [unwired: 1 in, 1 out]
          }
        }
      }
      frame "Error" {
        # "Error - Display an error dialog. This message is sent by the \"Error Handler\" VIs at the end of other loops in this application."
        n173 = Variant To Data(error in=w360, type=errorcluster {"status"=FALSE, "code"=0, "source"=""} ("error constant"), Variant=w358) -> (data=w356:errorcluster, error out=w355:errorcluster)
        n174 = call <vilib>:"Simple Error Handler.vi"("error in (no error)"=w356) -> ()  [unwired: 4 in, 5 out]
        n175 = Merge Errors(w355) -> (w354:errorcluster)
      }
      frame "Confirm Quit" {
        # "#CodeNeeded - If you want to provide an \"Are you sure\" dialog (or some other notification) before the application exits, place that code here. This message is typically sent from a Panel Close? event."
        # "Confirm Quit - Message that can confirm whether or not the user wants to exit the application."
        n176 = call-poly "Enqueue Message.vi"("Priority Message? (F)"=TRUE, "error in (no error)"=w367, "Message"="Exit", "Message Queue"=w363) -> ("error out"=w364:errorcluster)  [unwired: 6 in, 1 out]
        n177 = Merge Errors(w364) -> (w365:errorcluster)
      }
      frame "Exit" {
        w373 = FALSE  # Disable
        # "Exit - Exit the application."
        n178 = Unbundle By Name(w382) -> ("DAQ Mod ID"=w378:i32, "FCR Mod ID"=w372:i32)
        n179 = Release Queue(queue=w391, error in (no error)=w386) -> (error out=w374:errorcluster)  [unwired: 1 in, 2 out]
        n180 = Variant To Data(type=errorcluster {"status"=FALSE, "code"=0, "source"=""} ("error constant"), Variant=w383) -> (data=w384:errorcluster)  [unwired: 1 in, 1 out]
        n181 = call <vilib>:"Simple Error Handler.vi"("error in (no error)"=w384) -> ()  [unwired: 4 in, 5 out]
        n182 = call "Change disable state.vi"("error in"=w374, "Enter/Leave"=w373, "Address"=u8 1, "Module ID"=w372) -> ("error out"=w371:errorcluster)  [unwired: 7 in]
        n183 = call "wait -- subVI.vi"("error in (no error)"=w371) -> ("error out"=w370:errorcluster)  [unwired: 4 in]
        n184 = call "Change disable state.vi"("error in"=w370, "Enter/Leave"=w373, "Address"=u8 2, "Module ID"=w372) -> ("error out"=w369:errorcluster)  [unwired: 7 in]
        n185 = call "wait -- subVI.vi"("error in (no error)"=w369) -> ("error out"=w368:errorcluster)  [unwired: 4 in]
        n186 = call "Stop Module.vi"("error in"=w368, "Module ID"=w372) -> ("error out"=w377:errorcluster)  [unwired: 9 in]
        n187 = call "Stop task.vi"("error in"=w377, "Task list"=T12."All", "Module ID"=w378) -> ("error out"=w380:errorcluster)  [unwired: 8 in]
        n188 = call "Fire User Event - Stop.vi"("User Event - Stop"=w388) -> ("error out"=w387:errorcluster)  [unwired: 10 in]
        n189 = call "Stop Module.vi"("error in"=w380, "Module ID"=w378) -> ("error out"=w379:errorcluster)  [unwired: 9 in]
        n190 = Merge Errors(w387, w379) -> (w389:errorcluster)
      }
      frame Default {
        # "'Default' case only runs if there is a message that isn't defined in any of the other cases.  Output a programming error."
        n191 = xnode "Error Ring"("parameter 0"=w392) -> ("error out"=w393:errorcluster)
      }
    }
    n192 = call "Abeles-Brewster - Newport Error Handler - Message Handling Loop.vi"("error in (no error)"=w31, "Message Queue"=w30) -> ("dup error in"=w32:errorcluster)  [unwired: 8 in, 1 out]
  }
  n193 = while {
    tunnel: w27 -> [w408]
    shift-right: [w406] -> w23
    shift-left: w20 -> [w407]
    tunnel: [w402] -> w21
    stop <- w404 stop-if-true
    # "Event Handling Loop"
    n194 = event shown="[6] <NI DAQ Broadcast Events.Analog data acquired>: User Event" {
      selector: w407 -> [_ _ _ _ _ _ _ _ _ _ _ _ _ _ _ _ _ _ _ _ _]
      dyn-events: [_ _ _ _ _ _ _ _ _ _ _ _ _ _ _ _ _ _ _ _ _] -> w406
      timeout: _ -> [_ _ _ _ _ _ _ _ _ _ _ _ _ _ _ _ _ _ _ _ _]
      tunnel: [_ _ TRUE ("Discard?") _ _ _ _ _ _ _ _ _ _ _ _ _ _ _ _ _ _] -> w404
      tunnel: w408 -> [w413 w415 w417 w419 w430 w436 w442 w445 w454 w458 w462 w484 w487 w493 w498 w500 w507 w511 w515 w519 w524]
      tunnel: [w412 _ _ w420 w431 w434 w440 w443 w452 _ _ w482 w488 w492 w496 w501 w505 w509 w513 w517 w522] -> w405
      tunnel: [w411 w415 w417 w418 w428 w435 w441 w444 w453 w457 w462 w483 w485 w491 w497 w502 w506 w510 w514 w518 w523] -> w403
      event Panel Close? {
        # "Send the 'Confirm Quit' message if the user closes the panel of the VI. Discard the event so the 'Confirm Quit' message has a chance to run."
        n195 = event-data() -> ()  [unwired: 1 in, 1 out]
        n196 = call-poly "Enqueue Message.vi"("Priority Message? (F)"=TRUE, "Message"="Confirm Quit", "Message Queue"=w413) -> ("error out"=w412:errorcluster, "dup Message Queue"=w411:refnum<queue>)  [unwired: 7 in]
        n197 = event-data("Discard?"=TRUE) -> ()  [unwired: 1 in, 1 out]
      }
      event Application Instance Close {
        # "#CodeRecommended - When a project closes, all VIs within that project are aborted and leave memory. However, any code placed in this event frame is guaranteed to run to completion, so add any cleanup code that absolutely must happen here."
        n198 = event-data() -> ()  [unwired: 1 in, 1 out]
      }
      event User Event {
        # "The Message Handling Loop processed an \"Exit\" message, which fired this event to stop the Event Handling Loop."
        n199 = event-data() -> ()  [unwired: 1 in, 1 out]
      }
      event User Event {
        n200 = event-data() -> ()  [unwired: 1 in, 1 out]
        n201 = disable-structure shown="Disabled" {
          disable-tunnel: [w424 _] -> w420
          disable-tunnel: w419 -> [w423 w425]
          disable-tunnel: [w422 w425] -> w418
          frame Disabled {
            n202 = call-poly "Enqueue Message.vi"("Message"="Connect DAQ", "Message Queue"=w423) -> ("error out"=w424:errorcluster, "dup Message Queue"=w422:refnum<queue>)  [unwired: 8 in]
          }
          frame Enabled {
          }
        }
      }
      event User Event {
        n203 = event-data() -> ()  [unwired: 1 in, 1 out]
        n204 = call "Enqueue Message (Array).vi"("Message Data Array"=string[] ["", "DAQ Connected."], "Message Array"=string[] ["Connect FCR", "Update Display"] ("Message"), "Message Queue"=w430) -> ("error out"=w431:errorcluster, "dup Message Queue"=w428:refnum<queue>)  [unwired: 7 in]
        "DAQ Connected" <- TRUE ("DAQ Connected")
      }
      event User Event {
        n205 = event-data() -> ()  [unwired: 1 in, 1 out]
        n206 = call-poly "Enqueue Message.vi"("Message Data Array"=string[] ["Failed to connect to DAQ."] ("Message"), "Message Array"=string[] ["Update Display", "Call settings dialog"] ("Message"), "Message Queue"=w436) -> ("error out"=w434:errorcluster, "dup Message Queue"=w435:refnum<queue>)  [unwired: 7 in]
      }
      event User Event {
        n207 = event-data() -> ("Data"=w438:dbl[])  [unwired: 1 in]
        n208 = Index Array(array=w438) -> (element=w437:dbl)  [unwired: 1 in]
        n209 = call-poly "Enqueue Message.vi"("Message Data"=w437, "Message"="Update results", "Message Queue"=w442) -> ("error out"=w440:errorcluster, "dup Message Queue"=w441:refnum<queue>)  [unwired: 7 in]
      }
      event User Event {
        n210 = event-data() -> ()  [unwired: 1 in, 1 out]
        n211 = disable-structure shown="Enabled" {
          disable-tunnel: w445 -> [w449 w450]
          disable-tunnel: [w448 w450] -> w444
          disable-tunnel: [w447 _] -> w443
          frame Disabled {
            n212 = call-poly "Enqueue Message.vi"("Message"="Connect FCR", "Message Queue"=w449) -> ("error out"=w447:errorcluster, "dup Message Queue"=w448:refnum<queue>)  [unwired: 8 in]
          }
          frame Enabled {
          }
        }
      }
      event User Event {
        n213 = event-data() -> ()  [unwired: 1 in, 1 out]
        n214 = call "Enqueue Message (Array).vi"("Message Data Array"=string[] ["Connecting FCR..."], "Message Array"=string[] ["Update Display", "Validate connection"] ("Message"), "Message Queue"=w454) -> ("error out"=w452:errorcluster, "dup Message Queue"=w453:refnum<queue>)  [unwired: 7 in]
        "FCR Connected" <- TRUE ("FCR Connected")
      }
      event User Event {
        n215 = event-data() -> ()  [unwired: 1 in, 1 out]
        n216 = call-poly "Enqueue Message.vi"("Message Data Array"=string[] ["Failed to connect to FCR."] ("Message"), "Message Array"=string[] ["Update Display", "Call settings dialog"] ("Message"), "Message Queue"=w458) -> ("dup Message Queue"=w457:refnum<queue>)  [unwired: 7 in, 1 out]
      }
      event User Event {
        n217 = event-data() -> ("Module ID"=w461:i32, "State"=w464:T1, "Address"=w465:u8)  [unwired: 1 in]
        n218 = local read "Auto?"() -> (w463:bool)
        n219 = case shown="\"Ready\"" w464 {
          tunnel: w465 -> [_ w469]
          tunnel: w463 -> [_ w468]
          tunnel: w462 -> [_ w467]
          tunnel: w461 -> [_ w466]
          frame "Not referenced", Default {
          }
          frame "Ready" {
            n220 = case shown="False" w468 {
              tunnel: w469 -> [w473 _]
              tunnel: w467 -> [_ w479]
              tunnel: w466 -> [w472 _]
              frame False {
                # "Manual movement"
                n221 = case shown="2" w473 {
                  frame Default {
                  }
                  frame 1 {
                    w475 = T11."Enabled" ("Disabled")
                    n222 = local write "State 1"(Device_state_--_enum."Ready" ("State 1")) -> ()
                    n223 = property on="Inc platina 1" class="Bool"("DisabledEnum"=w475) -> ()  [unwired: 2 in, 2 out]
                    n224 = property on="Dec platina 1" class="Bool"("DisabledEnum"=w475) -> ()  [unwired: 2 in, 2 out]
                  }
                  frame 2 {
                    w477 = T11."Enabled" ("Disabled")
                    n225 = local write "State 2"(Device_state_--_enum."Ready" ("State 1")) -> ()
                    n226 = property on="Dec platina 2" class="Bool"("DisabledEnum"=w477) -> ()  [unwired: 2 in, 2 out]
                    n227 = property on="Inc platina 2" class="Bool"("DisabledEnum"=w477) -> ()  [unwired: 2 in, 2 out]
                  }
                }
                n228 = call "Get current position.vi"("Address"=u8 1, "Module ID"=w472) -> ("Position"=w470:dbl)  [unwired: 7 in, 2 out]
                n229 = local write "Curr angle"(w470) -> ()
              }
              frame True {
                # "Automatic movement."
                n230 = call-poly "Enqueue Message.vi"("Message"="End of acquisition", "Message Queue"=w479) -> ()  [unwired: 8 in, 2 out]
              }
            }
          }
        }
      }
      event User Event {
        n231 = event-data() -> ("Address"=w480:u8)  [unwired: 1 in]
        n232 = call-poly "Enqueue Message.vi"("Message Data"=w480, "Message"="Home reached", "Message Queue"=w484) -> ("error out"=w482:errorcluster, "dup Message Queue"=w483:refnum<queue>)  [unwired: 7 in]
      }
      event "Settings": Value Change {
        n233 = event-data() -> ()  [unwired: 1 in, 1 out]
        n234 = call-poly "Enqueue Message.vi"("Message"="Call settings dialog", "Message Queue"=w487) -> ("error out"=w488:errorcluster, "dup Message Queue"=w485:refnum<queue>)  [unwired: 8 in]
      }
      event "Exit": Value Change {
        n235 = event-data() -> ()  [unwired: 1 in, 1 out]
        n236 = call-poly "Enqueue Message.vi"("Priority Message? (F)"=TRUE, "Message"="Exit", "Message Queue"=w493) -> ("error out"=w492:errorcluster, "dup Message Queue"=w491:refnum<queue>)  [unwired: 7 in]
      }
      event "Controls.AutoMove.Home": Value Change {
        w494 = T11."Disabled and Grayed Out" ("Disabled")
        n237 = event-data() -> ()  [unwired: 1 in, 1 out]
        n238 = property on="AutoMove" class="Clust"("DisabledEnum"=w494) -> ()  [unwired: 2 in, 2 out]
        n239 = property on="ManMove" class="Clust"("DisabledEnum"=w494) -> ()  [unwired: 2 in, 2 out]
        n240 = property on="Refresh" class="Bool"("DisabledEnum"=w494) -> ()  [unwired: 2 in, 2 out]
        n241 = call-poly "Enqueue Message.vi"("Message"="Home", "Message Queue"=w498) -> ("error out"=w496:errorcluster, "dup Message Queue"=w497:refnum<queue>)  [unwired: 8 in]
      }
      event "Controls.AutoMove.Cancel": Value Change {
        n242 = event-data() -> ()  [unwired: 1 in, 1 out]
        n243 = call-poly "Enqueue Message.vi"("Message"="Stop movement", "Message Queue"=w500) -> ("error out"=w501:errorcluster, "dup Message Queue"=w502:refnum<queue>)  [unwired: 8 in]
      }
      event "Controls.ManMove.Inc platina 1", "Controls.ManMove.Dec platina 1", "Controls.ManMove.Inc platina 2", "Controls.ManMove.Dec platina 2": Value Change {
        n244 = event-data() -> ("CtlRef"=w503:refnum<vi>)  [unwired: 1 in]
        n245 = call-poly "Enqueue Message.vi"("Message Data"=w503, "Message"="Manual move", "Message Queue"=w507) -> ("error out"=w505:errorcluster, "dup Message Queue"=w506:refnum<queue>)  [unwired: 7 in]
      }
      event "Refresh": Value Change {
        n246 = event-data() -> ()  [unwired: 1 in, 1 out]
        n247 = call-poly "Enqueue Message.vi"("Message"="Update FCR parameters", "Message Queue"=w511) -> ("error out"=w509:errorcluster, "dup Message Queue"=w510:refnum<queue>)  [unwired: 8 in]
      }
      event "Controls.AutoMove.Move": Value Change {
        n248 = event-data() -> ()  [unwired: 1 in, 1 out]
        n249 = call-poly "Enqueue Message.vi"("Message"="Start aqcuisition", "Message Queue"=w515) -> ("error out"=w513:errorcluster, "dup Message Queue"=w514:refnum<queue>)  [unwired: 8 in]
      }
      event "Realizar Análisis": Value Change {
        n250 = event-data() -> ()  [unwired: 1 in, 1 out]
        n251 = call-poly "Enqueue Message.vi"("Message"="Analyze data", "Message Queue"=w519) -> ("error out"=w517:errorcluster, "dup Message Queue"=w518:refnum<queue>)  [unwired: 8 in]
      }
      event "Open File": Value Change {
        n252 = event-data() -> ("NewVal"=w520:path)  [unwired: 1 in]
        n253 = call-poly "Enqueue Message.vi"("Message Data"=w520, "Message"="Update range", "Message Queue"=w524) -> ("error out"=w522:errorcluster, "dup Message Queue"=w523:refnum<queue>)  [unwired: 7 in]
      }
    }
    n254 = call "Abeles-Brewster - Newport Error Handler - Event Handling Loop.vi"("error in (no error)"=w405, "Message Queue"=w403) -> ("dup error in"=w402:errorcluster)  [unwired: 8 in, 1 out]
  }
  n255 = Unregister For Events(event registration refnum=w23, error in=w21) -> (error out=w24:errorcluster)
  n256 = Merge Errors(w24, w28) -> (w25:errorcluster)
  n257 = call "Destroy User Event - Stop.vi"("error in (no error)"=w25, "User Event - Stop"=w19) -> ("error out"=w22:errorcluster)  [unwired: 9 in]
  n258 = disable-structure shown="Default" {
    disable-tunnel: w22 -> [_ _]
    frame condition #0 (active) {
    }
    frame condition #1 {
      # "Call Quit LabVIEW if running as a built application."
      n259 = Quit LabVIEW() -> ()  [unwired: 1 in]
    }
  }
